vi "Triangle Wave Generate text file.vi"() -> ()   [LabVIEW 2014]
uses:
  <vilib>/Utility/file.llb/Write To Spreadsheet File (I64).vi
panel:
  in  "distance between values":i32=1
  in  "file path (use dialog)":path
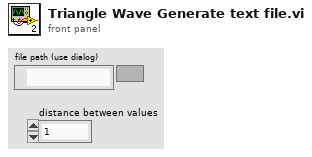
[diagram p1: front panel]
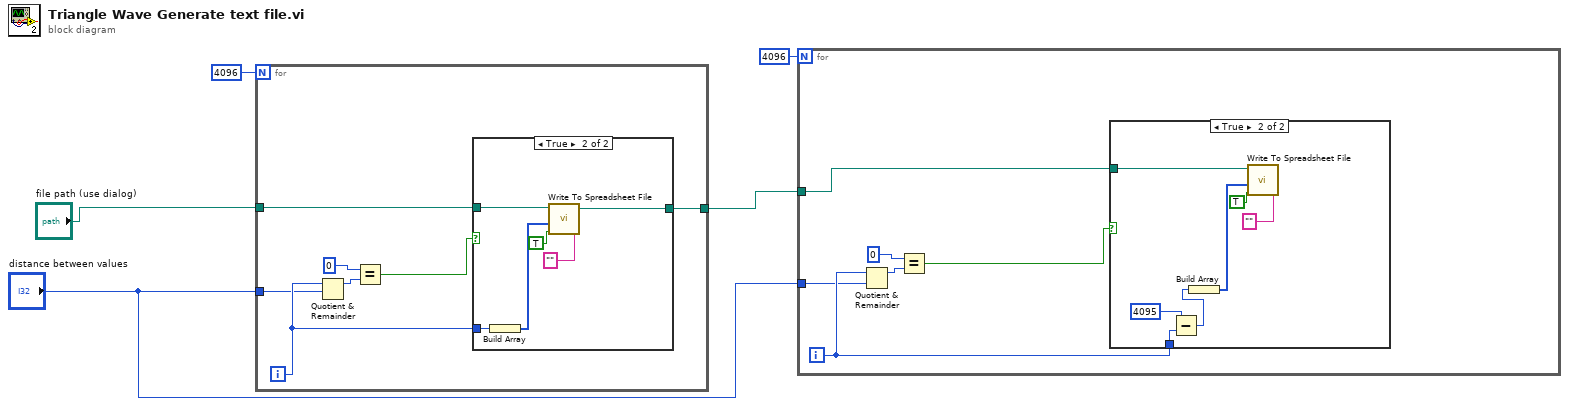
[diagram p0: block diagram]
diagram:
  n1 = for {
    N: 4096 -> [_]
    tunnel: "file path (use dialog)" -> [w11]
    tunnel: [w12] -> w2
    tunnel: "distance between values" -> [w6]
    i -> [w10]
    n2 = Quotient & Remainder(x=w10, y=w6) -> (x-y*floor(x/y)=w9:i32)  [unwired: 1 out]
    n3 = Equal?(x=0, y=w9) -> (x = y?=w7:bool)
    n4 = case shown="True" w7 {
      tunnel: w10 -> [_ w19]
      tunnel: w11 -> [w13 w16]
      tunnel: [w13 w14] -> w12
      frame False {
      }
      frame True {
        n5 = Build Array(w19) -> (w18:i32[])
        n6 = call-poly <vilib>:"Write To Spreadsheet File.vi"("delimiter (\\t)"="" ("delimiter (\\t)"), "append to file? (new file:F)"=TRUE, "1D data"=w18, "file path (dialog if empty)"=w16) -> ("new file path (Not A Path if cancelled)"=w14:path)  [unwired: 4 in]
      }
    }
  }
  n7 = for {
    N: 4096 -> [_]
    tunnel: w2 -> [w25]
    tunnel: "distance between values" -> [w20]
    i -> [w22]
    n8 = Quotient & Remainder(x=w22, y=w20) -> (x-y*floor(x/y)=w23:i32)  [unwired: 1 out]
    n9 = Equal?(x=0, y=w23) -> (x = y?=w21:bool)
    n10 = case shown="True" w21 {
      tunnel: w25 -> [_ w30]
      tunnel: w22 -> [_ w26]
      frame False {
      }
      frame True {
        n11 = Subtract(x=4095, y=w26) -> (x-y=w28:i32)
        n12 = Build Array(w28) -> (w32:i32[])
        n13 = call-poly <vilib>:"Write To Spreadsheet File.vi"("delimiter (\\t)"="" ("delimiter (\\t)"), "append to file? (new file:F)"=TRUE, "1D data"=w32, "file path (dialog if empty)"=w30) -> ()  [unwired: 4 in, 1 out]
      }
    }
  }
